vi "Test App Get Process Before Starting App.vi"(8 "error in (no error)":errorcluster, 11 "Rig Test in":refnum<class "Application Test.lvclass">) -> (0 "error out":errorcluster, 3 "Rig Test out":refnum<class "Application Test.lvclass">)   [LabVIEW 2020, in "Application Test.lvclass"]
uses:
  Application Test.lvclass
  <vilib>/Asteme/LUnit/Test Case.lvclass
  Framework/Application/Application.lvclass
  Framework/Process/Process.lvclass
  C:/Users/anton/Documents/GitHub/Triarc-Framework/source/Framework Test/Process Test/Process Test.lvclass
  C:/Users/anton/Documents/GitHub/Triarc-Framework/source/Framework Test/Base Class Test/Base Test.lvclass
  C:/Program Files (x86)/National Instruments/LabVIEW 2020/vi.lib/Asteme/LUnit/Test Case.lvclass
  C:/Users/anton/Documents/GitHub/Triarc-Framework/source/Framework Test/Application Test/Application Test.lvclass
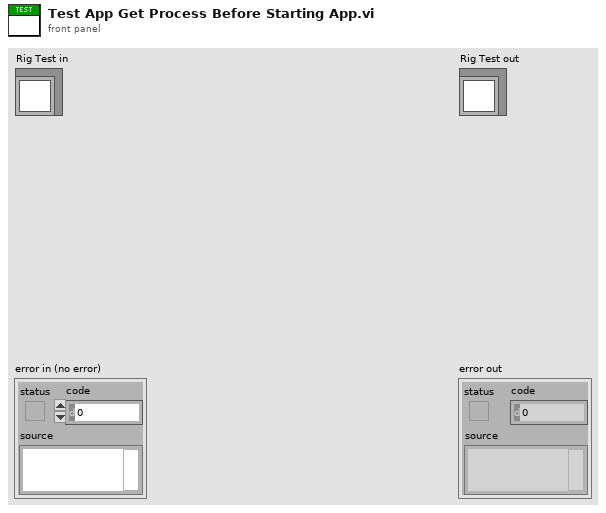
[diagram p1: front panel]
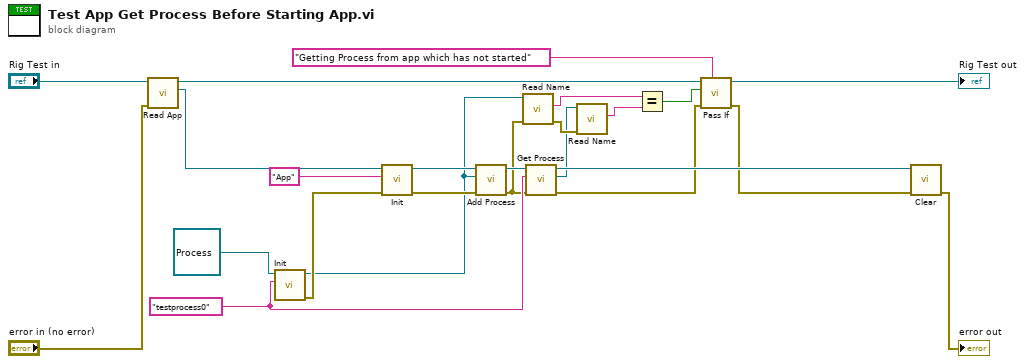
[diagram p0: block diagram]
diagram:
  w16 = "testprocess0" ("Name")
  n1 = call "Read App.vi"("error in (no error)"="error in (no error)", "Application Test In"="Rig Test in") -> ("App out"=w23:refnum<class "Application.lvclass">, "Application Test Out"=w15:refnum<class "Application Test.lvclass">)  [unwired: 7 in, 1 out]
  n2 = call-dynamic "Init.vi"("Name"=w16, "Process In"=refnum<class "Process.lvclass"> refnum ("Process.lvclass")) -> ("error out"=w10:errorcluster, "Process Out"=w5:refnum<class "Process.lvclass">)  [unwired: 8 in]
  n3 = call-dynamic "Init.vi"("error in (no error)"=w10, "Name"="App", "Process In"=w23) -> ("error out"=w18:errorcluster, "Process Out"=w20:refnum<class "Application.lvclass">)  [unwired: 7 in]
  n4 = call "Add Process.vi"("error in (no error)"=w18, "Process"=w5, "Rig In"=w20) -> ("error out"=w1:errorcluster, "Rig Out"=w21:refnum<class "Application.lvclass">)  [unwired: 7 in]
  n5 = call-dynamic "Read Name.vi"("error in (no error)"=w1, "Process In"=w5) -> ("error out"=w7:errorcluster, "Qualified Name"=w4:string)  [unwired: 6 in, 2 out]
  n6 = call "Get Process.vi"("error in (no error)"=w1, "Process Name"=w16, "Rig In"=w21) -> ("error out"=w11:errorcluster, "App Process"=w6:refnum<class "Process.lvclass">, "Rig Out"=w19:refnum<class "Application.lvclass">)  [unwired: 6 in]
  n7 = call-dynamic "Read Name.vi"("error in (no error)"=w7, "Process In"=w6) -> ("Qualified Name"=w3:string)  [unwired: 6 in, 3 out]
  n8 = Equal?(x=w4, y=w3) -> (x = y?=w2:bool)
  n9 = call <vilib>:"Pass If.vi"("Description"="Getting Process from app which has not started", "error in (no error)"=w11, "Pass?"=w2, "Test Case In"=w15) -> ("error out"=w12:errorcluster, "Test Case Out"=→"Rig Test out":refnum<class "Application Test.lvclass">)  [unwired: 6 in]
  n10 = call-dynamic "Clear.vi"("error in (no error)"=w12, "Application In"=w19) -> ("error out"=→"error out":errorcluster)  [unwired: 8 in, 1 out]
